vi "Extension Attributes.vi"() -> ()   [LabVIEW 2024]
uses:
  State Data.ctl
  <vilib>/Plug-In SDKs/Clients/Metadata/Hardware Item.ctl
  <vilib>/Plug-In SDKs/Clients/Metadata/Extension Value.ctl
  <vilib>/Plug-In SDKs/Clients/Data Store V1/Data Store Client.lvlibp/API/Data Store V1/Test Result.ctl
  <vilib>/Plug-In SDKs/Clients/Metadata/Outcome.ctl
  <vilib>/Plug-In SDKs/Clients/Metadata/Error Information.ctl
  <vilib>/Plug-In SDKs/Clients/Metadata/Step.ctl
  <vilib>/Plug-In SDKs/Clients/Metadata Store V1/Metadata Store Client.lvlibp/API/Metadata Store V1/Register Schema (Path).vi
  <vilib>/Plug-In SDKs/Clients/Metadata Store V1/Metadata Store Client.lvlibp/API/Metadata Store V1/Create Hardware Item.vi
  <vilib>/Plug-In SDKs/Clients/Data Store V1/Data Store Client.lvlibp/API/Data Store V1/Publish Measurement (DBL Analog Waveform).vi
  <vilib>/Plug-In SDKs/Clients/Data Store V1/Data Store Client.lvlibp/API/Data Store V1/Read Data from Measurement (DBL Analog Waveform).vi
  <vilib>/Plug-In SDKs/Clients/Metadata Store V1/Metadata Store Client.lvlibp
  <vilib>/Plug-In SDKs/Clients/Metadata/NI Metadata Types.lvlib
  <vilib>/Plug-In SDKs/Clients/Data Store V1/Data Store Client.lvlibp
  <vilib>/measure/NI_MABase.lvlib
panel:
  in  "schema file extension":enum16{"JSON", "TOML"}(ring)
  out "queried data":waveform(dbl)(graph)
  out "log":string
  out "error out":errorcluster
  # "Extension Attributes\n\nIn this example:\n- Create metadata entities with extension attributes.\n- Publish waveform data with metadata attached.\n- Query the measurement based on extension attributes."
  # "Schema files can be written in either JSON or TOML. This example includes both formats so you can compare them."
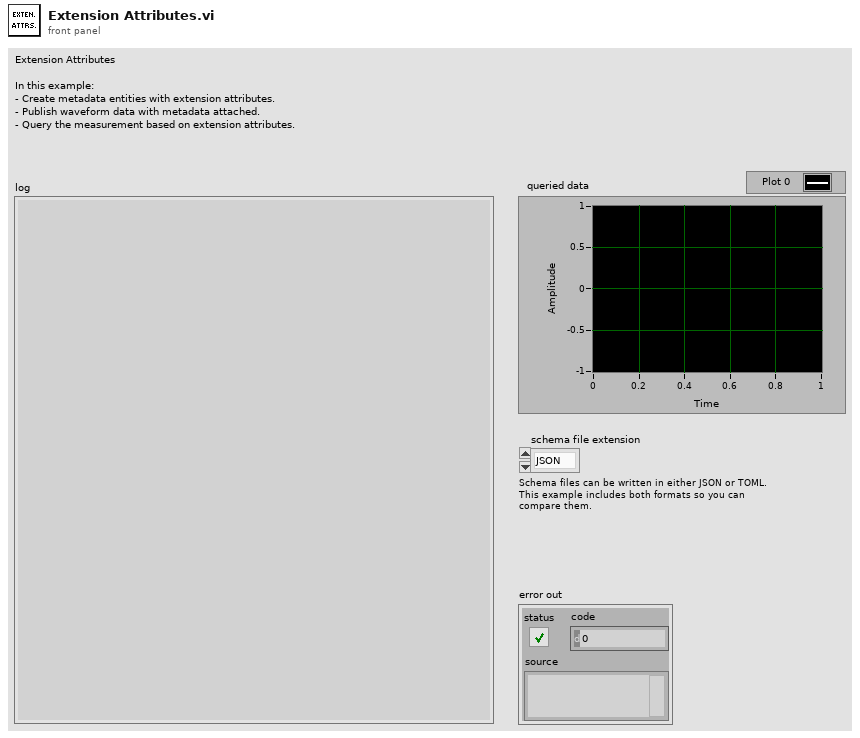
[diagram p1: front panel]
types:
  T1 = typedef "State Data.ctl" = cluster{"cable id":string, "socket id":string, "scope id":string, "test result id":string, "measurement name":string}
  T2 = enum16{"Create Cable", "Create Socket", "Create Scope", "Create Test Result", "Publish Measurement With Hardware", "Query Published Data"}
  T3 = typedef "Environment Values.ctl" = cluster{"cluster id":string, "failed ingest dir":string, "data files dir":string, "ingest dir":string, "db path":string, "cache expiration":string}
  T4 = typedef "NI Metadata Types.lvlib/Extension Value.ctl" = cluster{"name":string, "value":string}
  T5 = typedef "NI Metadata Types.lvlib/Hardware Item.ctl" = cluster{"model":string, "manufacturer":string, "part number":string, "serial number":string, "calibration due date":string, "asset identifier":string, "id":string, "link":string, "extension":T4[], "schema id":string}
  T6 = typedef "Data Store Client.lvlibp/Test Result.ctl" = cluster{"name":string, "start date time":timestamp, "end date time":timestamp, "outcome":T7, "error information":T8, "id":string, "uut instance id":string, "operator id":string, "test station id":string, "test description id":string, "software item ids":string[], "hardware item ids":string[], "test adapter ids":string[], "link":string, "extension":T4[], "schema id":string}
  T7 = typedef "NI Metadata Types.lvlib/Outcome.ctl" = enum32{"Unspecified", "Passed", "Failed", "Indeterminate"}
  T8 = typedef "NI Metadata Types.lvlib/Error Information.ctl" = cluster{"error code":i32, "message":string, "source":string}
  T9 = typedef "NI Metadata Types.lvlib/Step.ctl" = cluster{"name":string, "step type":string, "start date time":timestamp, "end date time":timestamp, "notes":string, "outcome":T7, "error information":T8, "id":string, "parent step id":string, "test result id":string, "test id":string, "link":string, "extension":T4[], "schema id":string}
  T10 = typedef "Data Store Client.lvlibp/Published Measurement.ctl" = cluster{"parametric index":i32, "name":string, "value type":string, "notes":string, "start date time":timestamp, "end date time":timestamp, "outcome":T7, "error information":T8, "published conditions":T11[], "data moniker":T12, "id":string, "test result id":string, "step id":string, "software item ids":string[], "hardware item ids":string[], "test adapter ids":string[]}
  T11 = typedef "Data Store Client.lvlibp/Published Condition.ctl" = cluster{"name":string, "condition type":string, "moniker":T12, "id":string, "step id":string, "test result id":string}
  T12 = typedef "Data Store Client.lvlibp/Data Moniker.ctl" = cluster{"service location":string, "data source":string, "data instance":i64}
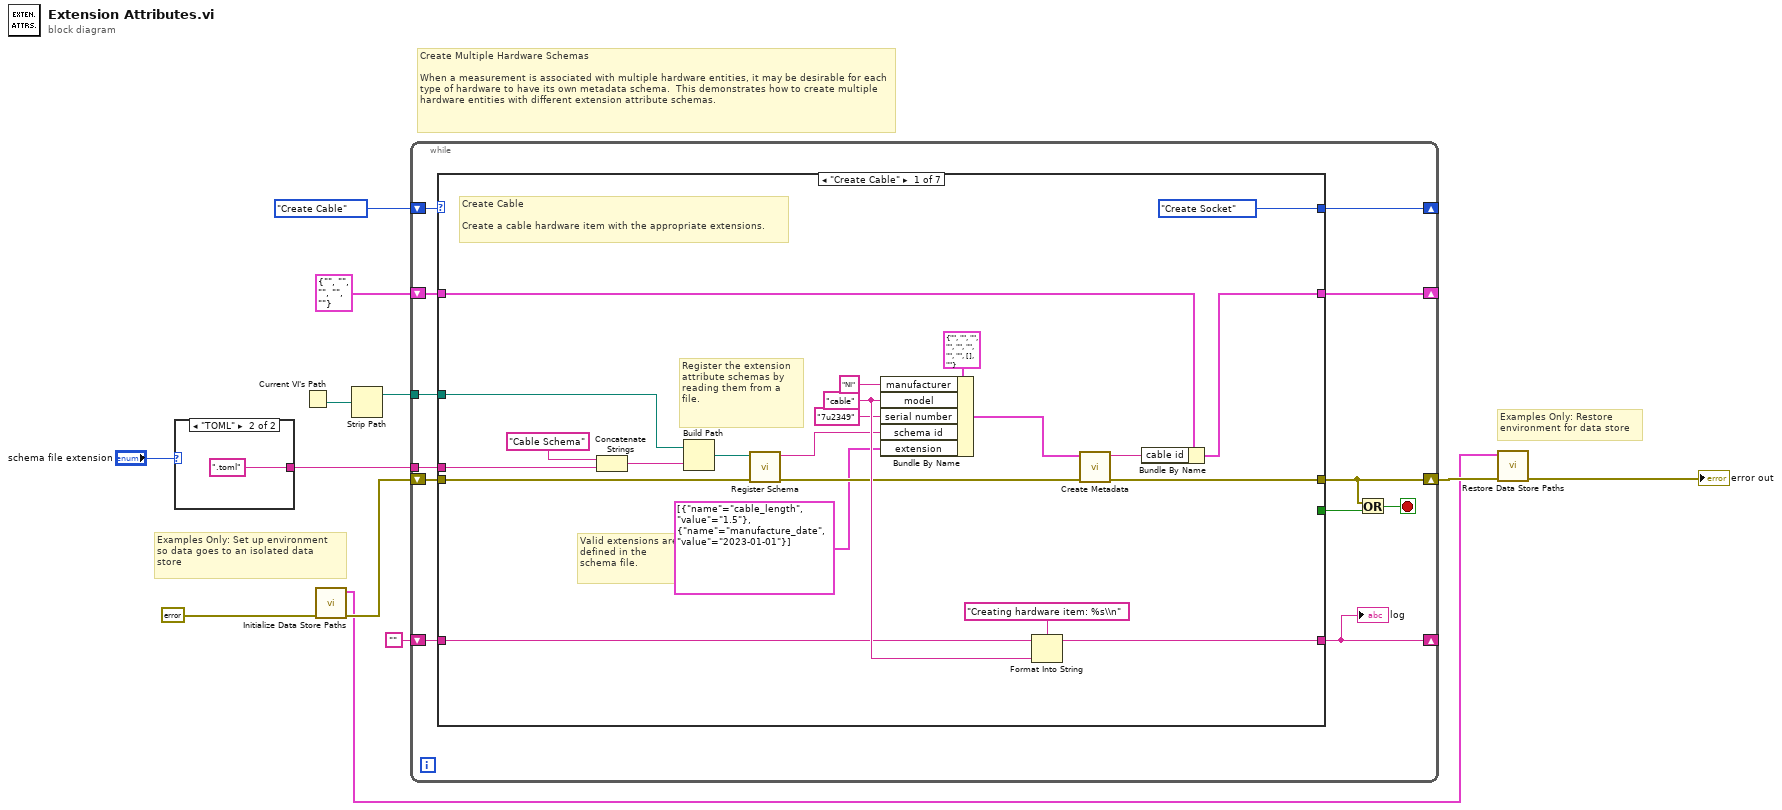
[diagram p0: block diagram]
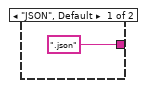
[diagram p2: hidden frame]
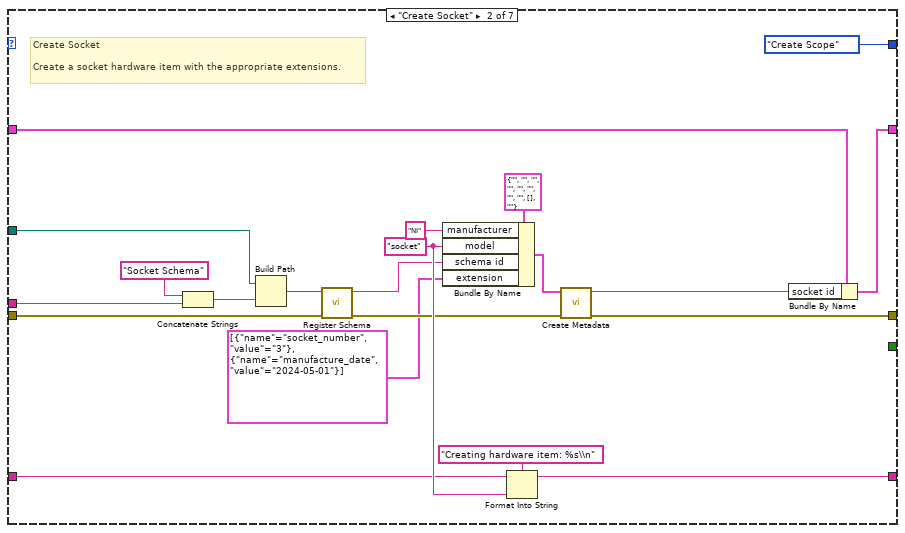
[diagram p3: hidden frame]
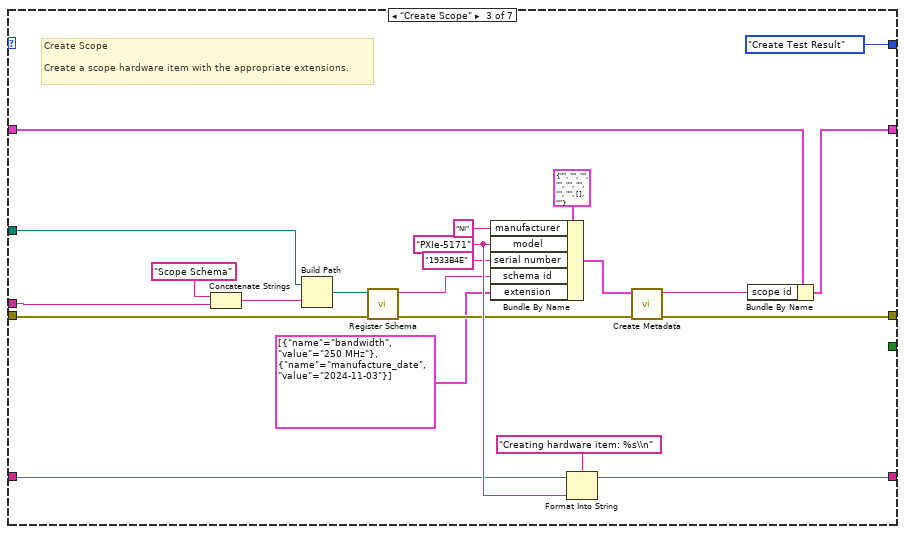
[diagram p4: hidden frame]
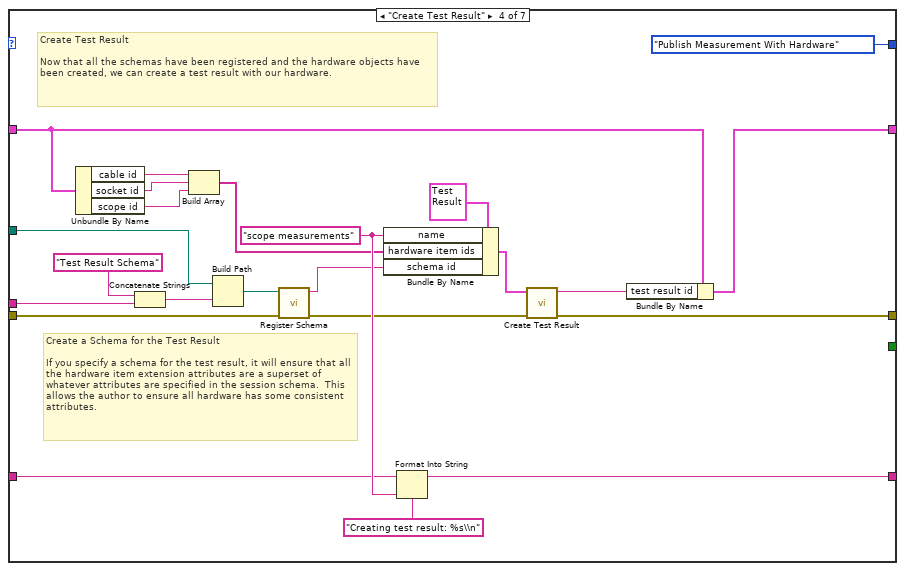
[diagram p5: hidden frame]
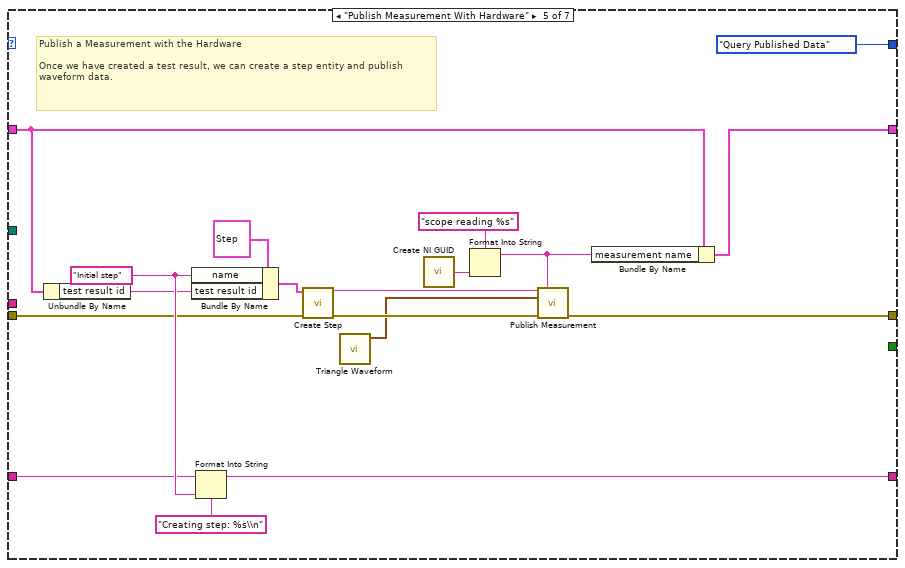
[diagram p6: hidden frame]
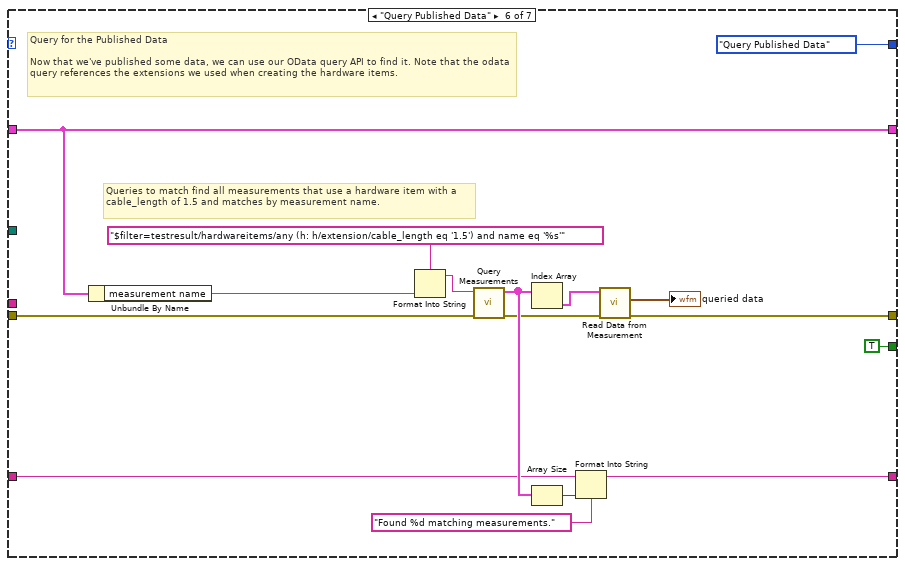
[diagram p7: hidden frame]
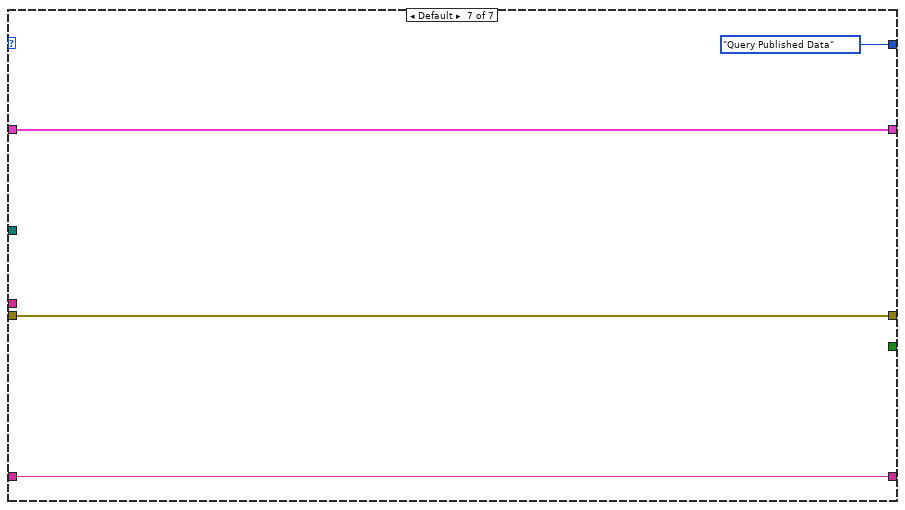
[diagram p8: hidden frame]
diagram:
  # "Examples Only: Restore\nenvironment for data store"
  # "Examples Only: Set up environment\nso data goes to an isolated data\nstore"
  # "Create Multiple Hardware Schemas\n\nWhen a measurement is associated with multiple hardware entities, it may be desirable for each type of hardware to have its own metadata schema.  This demonstrates how to create multiple hardware entities with different extension attribute schemas."
  n1 = case shown="\"TOML\"" "schema file extension" {
    tunnel: [".json" ("test result name") ".toml" ("test result name")] -> w7
    frame "JSON", Default {
    }
    frame "TOML" {
    }
  }
  n2 = Current VI's Path() -> (path=w10:path)
  n3 = call "Initialize Data Store Paths.vi"("error in"=errorcluster {"status"=FALSE, "code"=0, "source"=""} ("error out")) -> ("error out"=w4:errorcluster, "original values"=w2:T3)  [unwired: 9 in]
  n4 = Strip Path(path=w10) -> (stripped path=w9:path)  [unwired: 1 out]
  n5 = while {
    shift-right: [w18] -> w3
    shift-left: w4 -> [w25]
    shift-right: [w23] -> _
    shift-left: "" -> [w24]
    shift-right: [w15] -> _
    shift-left: T2."Create Cable" -> [w26]
    tunnel: w9 -> [w22]
    tunnel: w7 -> [w21]
    shift-right: [w16] -> _
    shift-left: T1 {"cable id"="", "socket id"="", "scope id"="", "test result id"="", "measurement name"=""} ("Cluster") -> [w17]
    stop <- w20 stop-if-true
    n6 = case shown="\"Create Cable\"" w26 {
      tunnel: [w30 w58 w73 w95 w120 w141 w151] -> w18
      tunnel: w25 -> [w37 w53 w79 w108 w123 w143 w151]
      tunnel: [w29 w59 w72 w94 w121 w140 w150] -> w23
      tunnel: w24 -> [w31 w51 w80 w110 w122 w142 w150]
      tunnel: [_ _ _ _ _ TRUE _] -> w19
      tunnel: w22 -> [w35 w54 w77 w105 _ _ _]
      tunnel: w21 -> [w36 w52 w78 w103 _ _ _]
      tunnel: w17 -> [w34 w57 w76 w97 w117 w135 w152]
      tunnel: [w32 w55 w74 w93 w118 w135 w152] -> w16
      tunnel: [T2."Create Socket" T2."Create Scope" T2."Create Test Result" T2."Publish Measurement With Hardware" T2."Query Published Data" T2."Query Published Data" T2."Query Published Data"] -> w15
      frame "Create Cable" {
        w48 = "cable" ("model")
        # "Create Cable\n\nCreate a cable hardware item with the appropriate extensions."
        # "Valid extensions are defined in the schema file."
        # "Register the extension attribute schemas by reading them from a file."
        n7 = Concatenate Strings("Cable Schema" ("test result name"), w36) -> (w39:string)
        n8 = Build Path(base path=w35, name or relative path=w39) -> (appended path=w41:path)
        n9 = call-poly <vilib>:"Register Schema.vi"("error in"=w37, "schema"=w41) -> ("error out"=w42:errorcluster, "schema id"=w40:string)  [unwired: 8 in]
        n10 = Bundle By Name(cluster=T5 {"model"="", "manufacturer"="", "part number"="", "serial number"="", "calibration due date"="", "asset identifier"="", "id"="", "link"="", "extension"=[], "schema id"=""} ("hardware item"), "manufacturer"="NI", "model"=w48, "serial number"="7u2349", "schema id"=w40, "extension"=T4[] [{"name"="cable_length", "value"="1.5"}, {"name"="manufacture_date", "value"="2023-01-01"}]) -> (w43:T5)
        n11 = Format Into String(format string="Creating hardware item: %s\\n", initial string=w31, w48) -> (resulting string=w29:string)  [unwired: 1 in, 1 out]
        n12 = call-poly <vilib>:"Create Metadata.vi"("error in"=w42, "hardware item"=w43) -> ("error out"=w30:errorcluster, "hardware item id"=w33:string)  [unwired: 8 in]
        n13 = Bundle By Name(cluster=w34, "cable id"=w33) -> (w32:T1)
      }
      frame "Create Socket" {
        w69 = "socket" ("socket model")
        # "Create Socket\n\nCreate a socket hardware item with the appropriate extensions."
        n14 = Concatenate Strings("Socket Schema" ("test result name"), w52) -> (w60:string)
        n15 = Build Path(base path=w54, name or relative path=w60) -> (appended path=w64:path)
        n16 = call-poly <vilib>:"Register Schema.vi"("error in"=w53, "schema"=w64) -> ("error out"=w63:errorcluster, "schema id"=w62:string)  [unwired: 8 in]
        n17 = Bundle By Name(cluster=T5 {"model"="", "manufacturer"="", "part number"="", "serial number"="", "calibration due date"="", "asset identifier"="", "id"="", "link"="", "extension"=[], "schema id"=""} ("hardware item"), "manufacturer"="NI" ("socket manufacturer"), "model"=w69, "schema id"=w62, "extension"=T4[] [{"name"="socket_number", "value"="3"}, {"name"="manufacture_date", "value"="2024-05-01"}]) -> (w66:T5)
        n18 = Format Into String(format string="Creating hardware item: %s\\n", initial string=w51, w69) -> (resulting string=w59:string)  [unwired: 1 in, 1 out]
        n19 = call-poly <vilib>:"Create Metadata.vi"("error in"=w63, "hardware item"=w66) -> ("error out"=w58:errorcluster, "hardware item id"=w56:string)  [unwired: 8 in]
        n20 = Bundle By Name(cluster=w57, "socket id"=w56) -> (w55:T1)
      }
      frame "Create Scope" {
        w91 = "PXIe-5171" ("model")
        # "Create Scope\n\nCreate a scope hardware item with the appropriate extensions."
        n21 = Concatenate Strings("Scope Schema" ("test result name"), w78) -> (w81:string)
        n22 = Build Path(base path=w77, name or relative path=w81) -> (appended path=w85:path)
        n23 = call-poly <vilib>:"Register Schema.vi"("error in"=w79, "schema"=w85) -> ("error out"=w84:errorcluster, "schema id"=w83:string)  [unwired: 8 in]
        n24 = Bundle By Name(cluster=T5 {"model"="", "manufacturer"="", "part number"="", "serial number"="", "calibration due date"="", "asset identifier"="", "id"="", "link"="", "extension"=[], "schema id"=""} ("scope"), "manufacturer"="NI", "model"=w91, "serial number"="1933B4E", "schema id"=w83, "extension"=T4[] [{"name"="bandwidth", "value"="250 MHz"}, {"name"="manufacture_date", "value"="2024-11-03"}]) -> (w88:T5)
        n25 = Format Into String(format string="Creating hardware item: %s\\n", initial string=w80, w91) -> (resulting string=w72:string)  [unwired: 1 in, 1 out]
        n26 = call-poly <vilib>:"Create Metadata.vi"("error in"=w84, "hardware item"=w88) -> ("error out"=w73:errorcluster, "hardware item id"=w75:string)  [unwired: 8 in]
        n27 = Bundle By Name(cluster=w76, "scope id"=w75) -> (w74:T1)
      }
      frame "Create Test Result" {
        w114 = "scope measurements" ("test result name")
        # "Create Test Result\n\nNow that all the schemas have been registered and the hardware objects have been created, we can create a test result with our hardware."
        # "Create a Schema for the Test Result\n\nIf you specify a schema for the test result, it will ensure that all the hardware item extension attributes are a superset of whatever attributes are specified in the session schema.  This allows the author to ensure all hardware has some consistent attributes."
        n28 = Unbundle By Name(w97) -> ("cable id"=w101:string, "socket id"=w99:string, "scope id"=w100:string)
        n29 = Concatenate Strings("Test Result Schema" ("test result name"), w103) -> (w104:string)
        n30 = Build Array(w101, w99, w100) -> (w98:string[])
        n31 = Build Path(base path=w105, name or relative path=w104) -> (appended path=w109:path)
        n32 = call-poly <vilib>:"Register Schema.vi"("error in"=w108, "schema"=w109) -> ("error out"=w107:errorcluster, "schema id"=w106:string)  [unwired: 8 in]
        n33 = Bundle By Name(cluster=T6 {"name"="", "start date time"=timestamp(0 s since 1904-01-01), "end date time"=timestamp(0 s since 1904-01-01), "outcome"=enum."Unspecified", "error information"={"error code"=0, "message"="", "source"=""}, "id"="", "uut instance id"="", "operator id"="", "test station id"="", "test description id"="", "software item ids"=[], "hardware item ids"=[], "test adapter ids"=[], "link"="", "extension"=[], "schema id"=""} ("test result"), "name"=w114, "hardware item ids"=w98, "schema id"=w106) -> (w111:T6)
        n34 = Format Into String(format string="Creating test result: %s\\n", initial string=w110, w114) -> (resulting string=w94:string)  [unwired: 1 in, 1 out]
        n35 = call <vilib>:"Create Test Result.vi"("error in"=w107, "test result"=w111) -> ("error out"=w95:errorcluster, "test result id"=w96:string)  [unwired: 8 in]
        n36 = Bundle By Name(cluster=w97, "test result id"=w96) -> (w93:T1)
      }
      frame "Publish Measurement With Hardware" {
        w131 = "Initial step" ("step name")
        # "Publish a Measurement with the Hardware\n\nOnce we have created a test result, we can create a step entity and publish waveform data."
        n37 = Unbundle By Name(w117) -> ("test result id"=w116:string)
        n38 = Bundle By Name(cluster=T9 {"name"="", "step type"="", "start date time"=timestamp(0 s since 1904-01-01), "end date time"=timestamp(0 s since 1904-01-01), "notes"="", "outcome"=enum."Unspecified", "error information"={"error code"=0, "message"="", "source"=""}, "id"="", "parent step id"="", "test result id"="", "test id"="", "link"="", "extension"=[], "schema id"=""} ("step"), "name"=w131, "test result id"=w116) -> (w128:T9)
        n39 = Format Into String(format string="Creating step: %s\\n", initial string=w122, w131) -> (resulting string=w121:string)  [unwired: 1 in, 1 out]
        n40 = call <vilib>:"Create Step.vi"("error in"=w123, "step"=w128) -> ("error out"=w126:errorcluster, "step id"=w127:string)  [unwired: 8 in]
        n41 = call <vilib>:"Triangle Waveform.vi"() -> ("signal out"=w125:waveform(dbl))  [unwired: 10 in, 1 out]
        n42 = call <vilib>:"Create NI GUID.vi"() -> ("NI GUID"=w124:string)
        n43 = Format Into String(format string="scope reading %s", w124) -> (resulting string=w119:string)  [unwired: 2 in, 1 out]
        n44 = call-poly <vilib>:"Publish Measurement.vi"("step id"=w127, "name"=w119, "waveform"=w125, "error in"=w126) -> ("error out"=w120:errorcluster)  [unwired: 9 in, 2 out]
        n45 = Bundle By Name(cluster=w117, "measurement name"=w119) -> (w118:T1)
      }
      frame "Query Published Data" {
        # "Query for the Published Data\n\nNow that we've published some data, we can use our OData query API to find it. Note that the odata query references the extensions we used when creating the hardware items."
        # "Queries to match find all measurements that use a hardware item with a cable_length of 1.5 and matches by measurement name."
        n46 = Unbundle By Name(w135) -> ("measurement name"=w136:string)
        n47 = Format Into String(format string="$filter=testresult/hardwareitems/any (h: h/extension/cable_length eq '1.5') and name eq '%s'" ("odata query"), w136) -> (resulting string=w137:string)  [unwired: 2 in, 1 out]
        n48 = call <vilib>:"Query Measurements.vi"("error in"=w143, "odata query"=w137) -> ("error out"=w144:errorcluster, "published measurements"=w146:T10[])  [unwired: 8 in]
        n49 = Index Array(array=w146) -> (element=w145:T10)  [unwired: 1 in]
        n50 = Array Size(array=w146) -> (size(s)=w148:i32)
        n51 = Format Into String(format string="Found %d matching measurements.", initial string=w142, w148) -> (resulting string=w140:string)  [unwired: 1 in, 1 out]
        n52 = call-poly <vilib>:"Read Data from Measurement.vi"("error in"=w144, "published measurement"=w145) -> ("error out"=w141:errorcluster, "waveform data"=→"queried data":waveform(dbl))  [unwired: 7 in, 1 out]
      }
      frame Default {
      }
    }
    "log" <- w23
    n53 = Or(x=w18, y=w19) -> (x .or. y?=w20:bool)
  }
  n54 = call "Restore Data Store Paths.vi"("error in"=w3, "original values"=w2) -> ("error out"=→"error out":errorcluster)  [unwired: 9 in]
